vi "NavigateToString.vi"(0 "reference in":refnum<class "LcWebView.lvclass">, 1 "HTML Content":string, 5 "Error In":errorcluster) -> (14 "reference out":refnum<class "LcWebView.lvclass">, 15 "Loaded":bool, 19 "Error Out":errorcluster)   [LabVIEW 2019, in "LcWebView.lvclass"]
doc: "Load dynamic HTML as string"
uses:
  LcWebView.lvclass
  D:/GitProjects/Public/GitHub/LcWebView/data/Microsoft.Web.WebView2.Core.dll
  data/Microsoft.Web.WebView2.Core.dll
panel:
  out "Status":i32(ring) items=["Created", "WaitingForActivation", "WaitingToRun", "Running", "WaitingForChildrenToComplete", "RanToCompletion", "Canceled", "Faulted"]
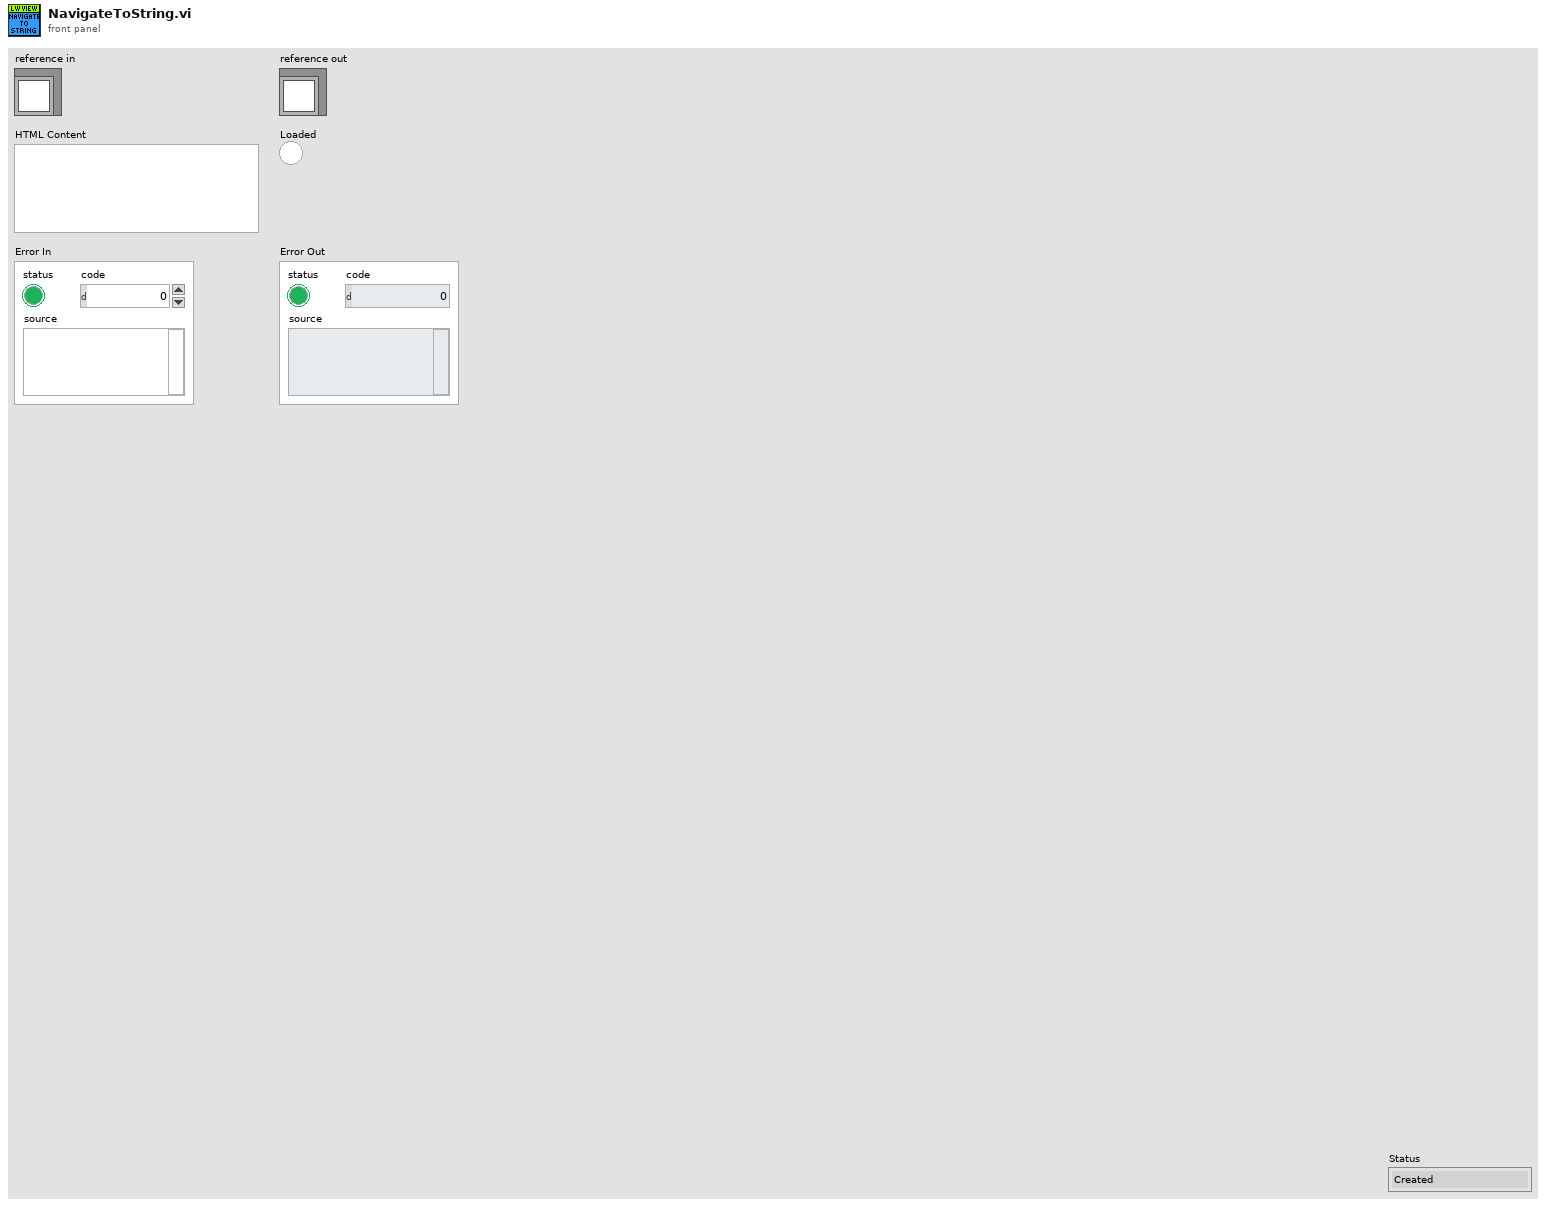
[diagram p1: front panel]
types:
  T1 = typedef "LcWebView.lvclass/ObjectAttributes.ctl" = cluster{"WebView Container":refnum<k24>, "CoreWebViewRef":refnum<k24>, "Status":i32, "Status Message":string, "User Data Folder":path, "BrowserProcessId":u32, "PlotMap":T2, "PlotType":T4}
  T2 = typedef "LcWebView.lvclass/PlotMap.ctl" = map{string, T3}
  T3 = typedef "LcWebView.lvclass/PlotRef.ctl" = cluster{"PlotType":T4, "PlotTemplate":string}
  T4 = typedef "LcWebView.lvclass/PlotType.ctl" = enum16{"bar", "line", "pie"}
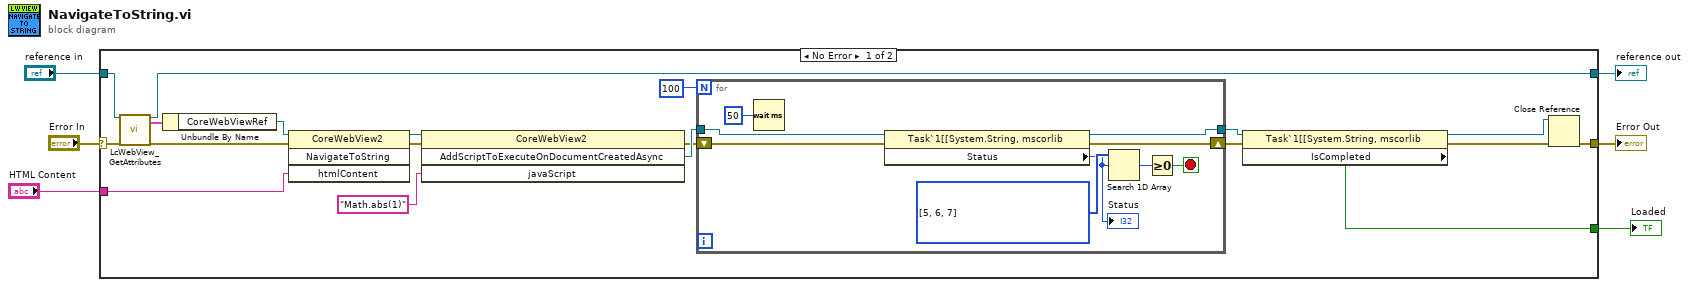
[diagram p0: block diagram]
diagram:
  n1 = case shown="No Error" "Error In" {
    selector: "Error In" -> [w25 w36]
    tunnel: [w8 w36] -> w5
    tunnel: [w23 w35] -> w3
    tunnel: "reference in" -> [w24 w35]
    tunnel: "HTML Content" -> [w19 _]
    tunnel: [w7 _] -> w1
    frame No Error {
      n2 = call "LcWebView_GetAttributes.vi"("reference in"=w24, "error in (no error)"=w25) -> ("reference out"=w23:refnum<class "LcWebView.lvclass">, "Data"=w22:T1, "error out"=w20:errorcluster)  [unwired: 14 in, 1 out]
      n3 = Unbundle By Name(w22) -> ("CoreWebViewRef"=w21:refnum<k24>)
      n4 = invoke class="CoreWebView2" method="NavigateToString"(reference=w21, error in=w20, "htmlContent"=w19) -> (reference out=w18:refnum<k24>, error out=w17:errorcluster)  [unwired: 1 in, 2 out]
      n5 = invoke class="CoreWebView2" method="AddScriptToExecuteOnDocumentCreatedAsync"(reference=w18, error in=w17, "javaScript"="Math.abs(1)") -> (error out=w14:errorcluster, "AddScriptToExecuteOnDocumentCreatedAsync"=w15:refnum<k24>)  [unwired: 1 in, 2 out]
      n6 = for {
        N: 100 -> [_]
        tunnel: w15 -> [w34]
        shift-right: [w32] -> w11
        shift-left: w14 -> [w33]
        tunnel: [w30] -> w12
        stop <- w26 stop-if-true
        w29 = i32[] [5, 6, 7] items=["Created", "WaitingForActivation", "WaitingToRun", "Running", "WaitingForChildrenToComplete", "RanToCompletion", "Canceled", "Faulted"] ("Status")
        n7 = Wait (ms)(milliseconds to wait=u32 50) -> ()  [unwired: 1 out]
        n8 = property class="Task`1[[System.String, mscorlib"(reference=w34, error in=w33) -> (reference out=w30:refnum<k24>, error out=w32:errorcluster, "Status"=w28:i32)
        "Status" <- w28
        n9 = Search 1D Array(1D array=w29, element=w28) -> (index of element=w27:i32)  [unwired: 1 in]
        n10 = Greater Or Equal To 0?(x=w27) -> (x >= 0?=w26:bool)
      }
      n11 = property class="Task`1[[System.String, mscorlib"(reference=w12, error in=w11) -> (reference out=w10:refnum<k24>, error out=w9:errorcluster, "IsCompleted"=w7:bool)
      n12 = Close Reference(reference=w10, error in (no error)=w9) -> (error out=w8:errorcluster)
    }
    frame Error {
    }
  }
  "Error Out" <- w5
  "reference out" <- w3
  "Loaded" <- w1
